vi "Find Workspace.vi"(6 "Pickup_Test_Number":dbl, 7 "Database Entry in":refnum<class "Database Entry.lvclass">, 8 "Error In":errorcluster, 9 "Assembly Type":string, 10 "Control In":T2={"I-O.lvclass"=refnum, "Gantry"=refnum, "Dispenser"="COM1"}, 11 "Carrier Tray in":refnum<class "Assembly Tray.lvclass">) -> (0 "Error Out":errorcluster, 1 "Workspace":T1, 2 "Control Out":T2={"I-O.lvclass"=refnum, "Gantry"=refnum, "Dispenser"="COM1"}, 3 "Carrier Tray Out":refnum<class "Assembly Tray.lvclass">, 5 "Database Entry out":refnum<class "Database Entry.lvclass">)   [LabVIEW 2021, in "Assembly Tray.lvclass"]
uses:
  Assembly Tray.lvclass
  C:/Users/HEP/Documents/GitHub/Gantry/UCSB-Gantry-HEP-main/Classes/Workspace/Fixture.lvclass
  Controller/Controllers.ctl
  Controller/I-O/I-O.lvclass
  C:/Program Files (x86)/Aerotech/A3200/LabVIEW/2010/Bin/Aerotech.A3200.dll
  Program Files (x86)/Aerotech/A3200/LabVIEW/2010/Bin/Aerotech.A3200.dll
  Workspace.ctl
  Assembly/Database Entry/Database Entry.lvclass
  Fixture.lvclass/Fixture.ctl
  Assembly Tray.lvclass/Assembly Tray.ctl
  Read Fixture ID.vi
  Read Position.vi
  Fixture.lvclass
  Controller/Controller.lvclass
panel:
  out "XYZTheta Centers":dbl[][](array[numeric])
  in  "output cluster 2":T1
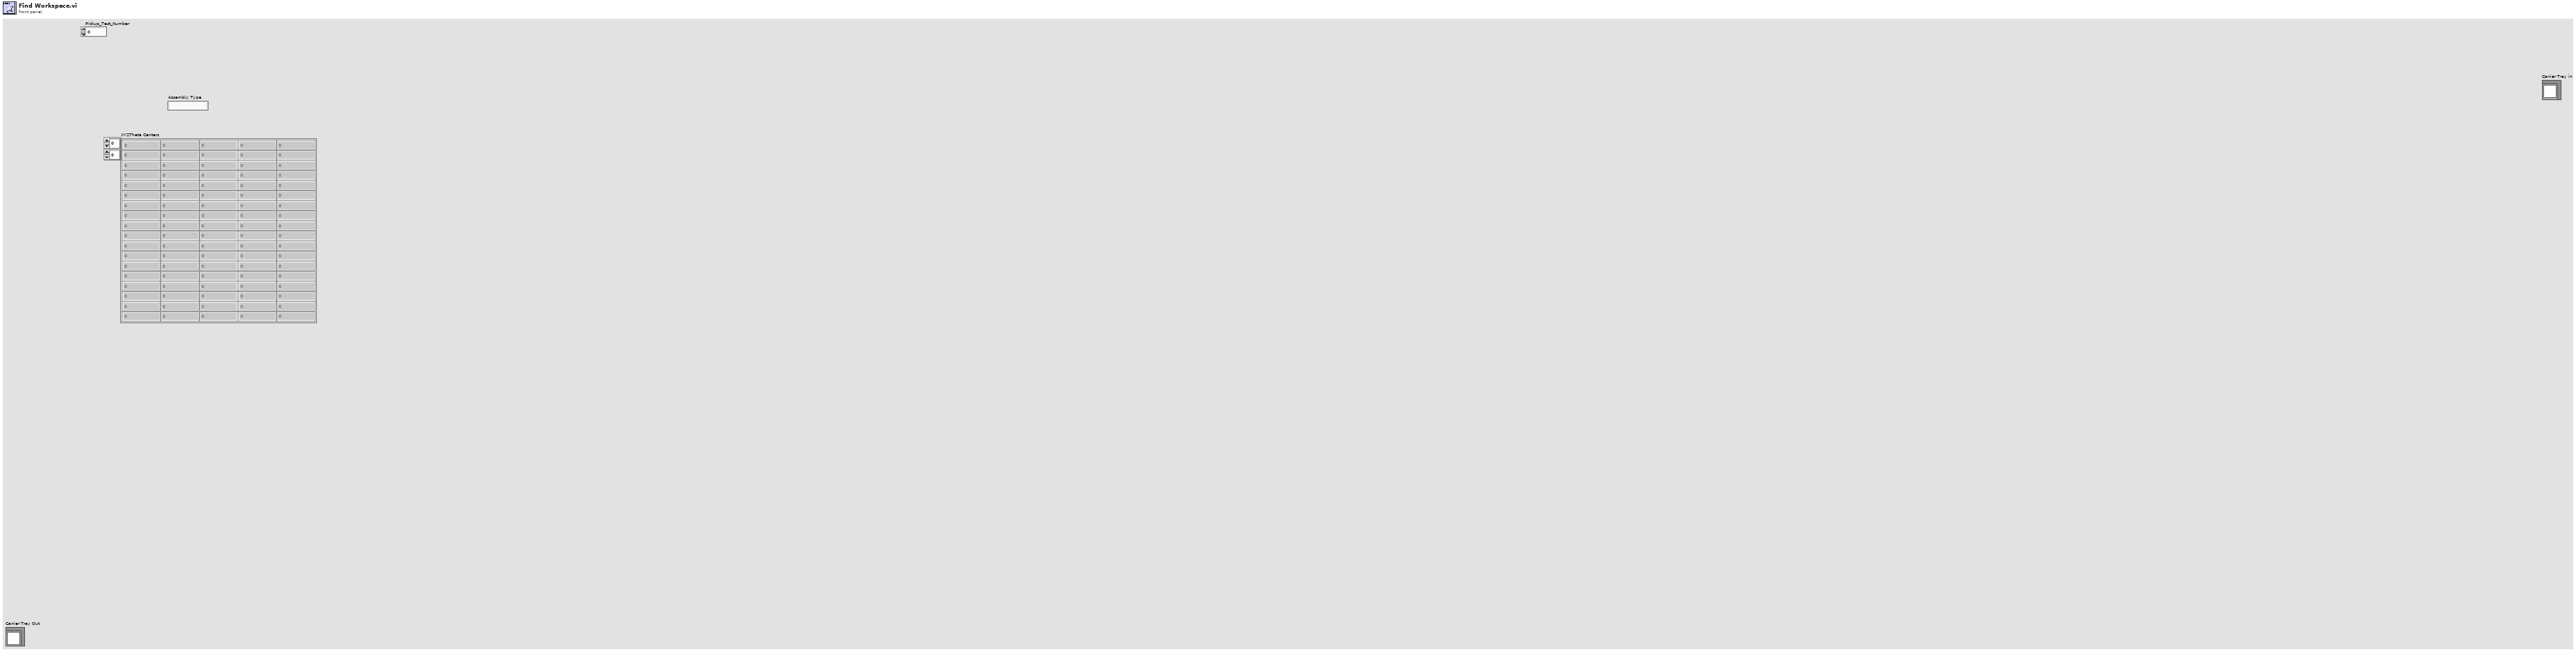
[diagram p1: front panel]
types:
  T1 = typedef "Fixture.lvclass/Workspace.ctl" = cluster{"XYZTheta":dbl[], "Workspace Valve":i32, "Workspace Sensor":i32, "Tray Number":i32, "Position":i32, "Assembly Type":string, "Numeric":dbl, "First Pos":i32}
  T2 = typedef "Controller.lvclass/Controllers.ctl" = cluster{"I-O.lvclass":refnum<class "I-O.lvclass">, "Gantry":refnum<k24>, "Dispenser":refnum<visa-resource-name>}
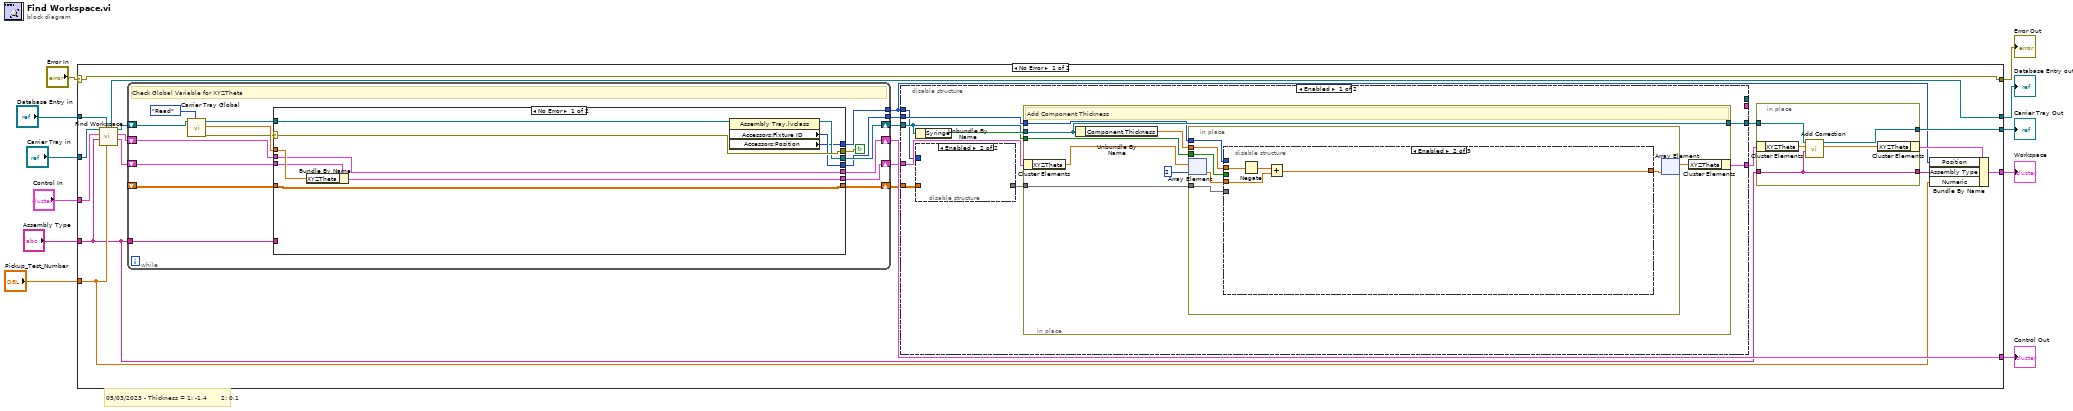
[diagram p0: block diagram]
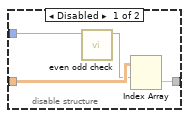
[diagram p2: hidden frame]
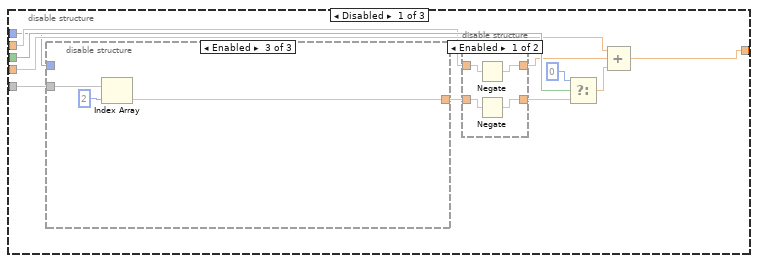
[diagram p3: hidden frame]
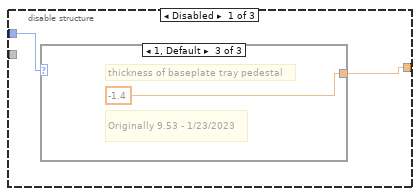
[diagram p4: hidden frame]
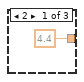
[diagram p5: hidden frame]
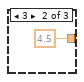
[diagram p6: hidden frame]
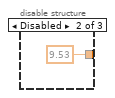
[diagram p7: hidden frame]
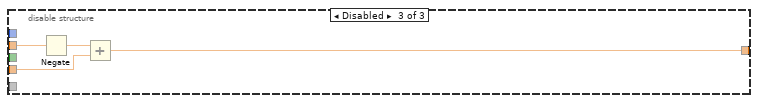
[diagram p9: hidden frame]
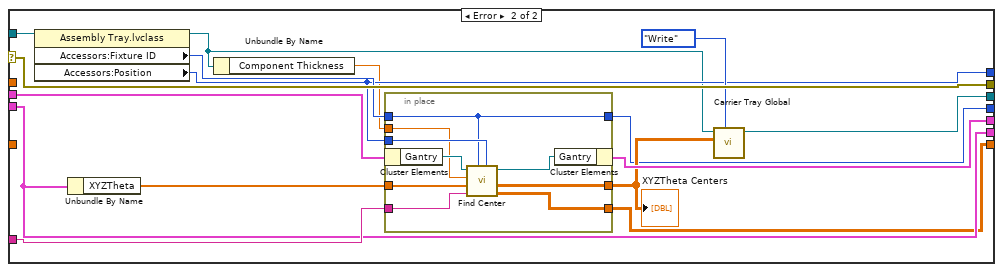
[diagram p11: hidden frame]
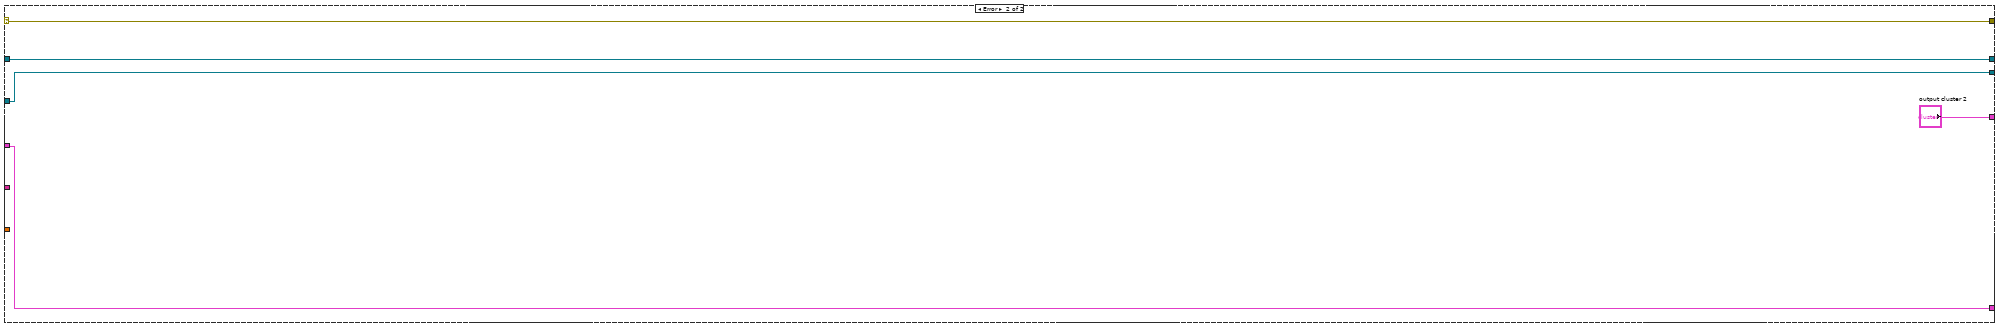
[diagram p12: hidden frame]
diagram:
  # "05/03/2023 - Thickness = 1: -1.4       2: 0.1"
  n1 = case shown="No Error" "Error In" {
    selector: "Error In" -> [w33 w156]
    tunnel: [w33 w156] -> w10
    tunnel: "Control In" -> [w32 w157]
    tunnel: [w30 w157] -> w8
    tunnel: "Carrier Tray in" -> [w31 w154]
    tunnel: [w18 "output cluster 2"] -> w6
    tunnel: [w20 w154] -> w5
    tunnel: "Assembly Type" -> [w12 _]
    tunnel: "Pickup_Test_Number" -> [w15 _]
    tunnel: "Database Entry in" -> [w14 w153]
    tunnel: [w13 w153] -> w1
    frame No Error {
      n2 = call-parent "Find Workspace.vi"("Pickup_Test_Number"=w15, "Database Entry in"=w14, "Assembly Type"=w12, "Control In"=w32, "Workspace In"=w31) -> (1:"Workspace Out"=w29:T1, "Control Out"=w28:T2, 3:"Workspace Out"=w25:refnum<class "Assembly Tray.lvclass">, "Database Entry out"=w13:refnum<class "Database Entry.lvclass">)  [unwired: 2 in, 1 out]
      n3 = while {
        shift-right: [w110] -> w27
        shift-left: w25 -> [w108]
        shift-right: [w112] -> w30
        shift-left: w28 -> [w113]
        shift-right: [w109] -> w26
        shift-left: w29 -> [w114]
        tunnel: w12 -> [w106]
        tunnel: [w105] -> w24
        shift-right: [w104] -> w23
        shift-left: _ -> [w103]
        tunnel: [w102] -> w16
        stop <- w116 continue-if-true
        # "Check Global Variable for XYZTheta"
        n4 = call "Carrier Tray Global.vi"("Action"=enum16{"Initialize", "Read", "Write"}."Read", "Carrier Tray.lvclass"=w108) -> ("error out"=w107:errorcluster, "XYZTheta out"=w115:dbl[], "Carrier Tray.lvclass 2"=w111:refnum<class "Assembly Tray.lvclass">)  [unwired: 7 in]
        n5 = case shown="No Error" w107 {
          selector: w107 -> [w127 w143]
          tunnel: [w127 w143] -> w116
          tunnel: w115 -> [w126 _]
          tunnel: [w125 w132] -> w109
          tunnel: w114 -> [w124 w132]
          tunnel: w113 -> [w123 w138]
          tunnel: [w123 w137] -> w112
          tunnel: w111 -> [w122 w140]
          tunnel: [w121 w142] -> w110
          tunnel: w106 -> [_ w134]
          tunnel: [w120 w133] -> w105
          tunnel: [w119 w131] -> w104
          tunnel: w103 -> [w119 _]
          tunnel: [w118 w130] -> w102
          frame No Error {
            n6 = Bundle By Name(cluster=w124, "XYZTheta"=w126) -> (w125:T1)
            n7 = property class="Assembly Tray.lvclass"(reference=w122) -> (reference out=w121:refnum<class "Assembly Tray.lvclass">, "Accessors:Fixture ID"=w120:i32, "Accessors:Position"=w118:i32)  [unwired: 1 in, 1 out]
          }
          frame Error {
            n8 = property class="Assembly Tray.lvclass"(reference=w140) -> (reference out=w129:refnum<class "Assembly Tray.lvclass">, "Accessors:Fixture ID"=w139:i32, "Accessors:Position"=w130:i32)  [unwired: 1 in, 1 out]
            n9 = Unbundle By Name(w132) -> ("XYZTheta"=w136:dbl[])
            n10 = Unbundle By Name(w129) -> ("Component Thickness"=w128:dbl)
            n11 = in-place {
              in-place-border: w139 -> [w146]
              in-place-border: w136 -> [w150]
              in-place-border: [w149] -> w135
              in-place-border: w134 -> [w148]
              in-place-border: w130 -> [w147]
              in-place-border: [w146] -> w133
              in-place-border: [w145] -> w131
              in-place-border: w128 -> [w144]
              n12 = in-place-cluster #1(w138) -> ("Gantry"=w152:refnum<k24>)
              n13 = call "Find Center.vi"("Position"=w147, "Tray Number"=w146, "Assembly Type"=w148, "XYZTheta"=w150, "component thickness"=w144, "Gantry In"=w152) -> ("Pedestal Heights"=w145:dbl[][], "XYZTheta Centers"=w149:dbl[][], "Gantry Out"=w151:refnum<k24>)  [unwired: 3 in]
              n14 = in-place-cluster #1("Gantry"=w151) -> (w137:T2)
            }
            "XYZTheta Centers" <- w135
            n15 = call "Carrier Tray Global.vi"("Action"=enum16{"Initialize", "Read", "Write"}."Write", "XYZTheta in"=w135, "Carrier Tray.lvclass"=w129) -> ("Carrier Tray.lvclass 2"=w142:refnum<class "Assembly Tray.lvclass">)  [unwired: 6 in, 2 out]
          }
        }
      }
      n16 = disable-structure shown="Enabled" {
        disable-tunnel: [_ w100] -> _
        disable-tunnel: [_ w101] -> _
        disable-tunnel: w27 -> [w47 w100]
        disable-tunnel: w26 -> [w46 w101]
        disable-tunnel: w24 -> [w44 _]
        disable-tunnel: w23 -> [w41 _]
        disable-tunnel: [w43 _] -> w22
        disable-tunnel: [w42 _] -> w21
        disable-tunnel: w16 -> [w39 _]
        frame Enabled {
          n17 = Unbundle By Name(w47) -> ("Syringe"=w45:bool)
          n18 = disable-structure shown="Enabled" {
            disable-tunnel: w41 -> [w51 _]
            disable-tunnel: [w50 _] -> w40
            disable-tunnel: w39 -> [w48 _]
            frame Disabled {
              n19 = call "even odd check.vi"("position"=w48) -> ("index"=w49:i32)  [unwired: 10 in]
              n20 = Index Array(array=w51, index (row)=w49) -> (element=w50:dbl[])  [unwired: 1 in]
            }
            frame Enabled {
            }
          }
          n21 = in-place {
            in-place-border: w47 -> [w57]
            in-place-border: [w57] -> w42
            in-place-border: w45 -> [w56]
            in-place-border: w44 -> [w54]
            in-place-border: w40 -> [w52]
            # "Add Component Thickness"
            n22 = in-place-cluster #2(w46) -> ("XYZTheta"=w55:dbl[])
            n23 = Unbundle By Name(w57) -> ("Component Thickness"=w58:dbl)
            n24 = in-place {
              in-place-border: w58 -> [w62]
              in-place-border: w56 -> [w64]
              in-place-border: w54 -> [w61]
              in-place-border: w52 -> [w60]
              n25 = in-place-array #3(w55, 2) -> (w63:dbl)
              n26 = disable-structure shown="Enabled" {
                disable-tunnel: [w76 w94 w98] -> w65
                disable-tunnel: w64 -> [w75 _ _]
                disable-tunnel: w63 -> [w72 w95 w99]
                disable-tunnel: w62 -> [w71 w93 w97]
                disable-tunnel: w61 -> [w67 _ _]
                disable-tunnel: w60 -> [w66 _ _]
                frame Disabled {
                  n27 = disable-structure shown="Enabled" {
                    disable-tunnel: [w78 9.53 w85] -> w69
                    disable-tunnel: w67 -> [w77 _ _]
                    disable-tunnel: w66 -> [_ _ w84]
                    frame Disabled {
                      n28 = case shown="1, Default" w77 {
                        tunnel: [4.4 4.5 -1.4] -> w78
                        frame 2 {
                        }
                        frame 3 {
                        }
                        frame 1, Default {
                          # "thickness of baseplate tray pedestal"
                          # "Originally 9.53 - 1/23/2023"
                        }
                      }
                    }
                    frame Disabled {
                    }
                    frame Enabled {
                      n29 = Index Array(array=w84, index=2) -> (element=w85:dbl)
                    }
                  }
                  n30 = disable-structure shown="Enabled" {
                    disable-tunnel: w71 -> [w89 w91]
                    disable-tunnel: [w88 w91] -> w70
                    disable-tunnel: w69 -> [w87 w90]
                    disable-tunnel: [w86 w90] -> w68
                    frame Enabled {
                      n31 = Negate(x=w89) -> (-x=w88:dbl)
                      n32 = Negate(x=w87) -> (-x=w86:dbl)
                    }
                    frame Disabled {
                    }
                  }
                  n33 = Select(t=0, s=w75, f=w68) -> (s? t:f=w73:dbl)
                  n34 = Compound Arithmetic op=ADD(w72, w70, w73) -> (w76:dbl)
                }
                frame Enabled {
                  n35 = Negate(x=w93) -> (-x=w92:dbl)
                  n36 = Add(x=w92, y=w95) -> (x+y=w94:dbl)
                }
                frame Disabled {
                  n37 = Negate(x=w97) -> (-x=w96:dbl)
                  n38 = Add(x=w96, y=w99) -> (x+y=w98:dbl)
                }
              }
              n39 = in-place-array #3(w65) -> (w59:dbl[])  [unwired: 1 out]
            }
            n40 = in-place-cluster #2("XYZTheta"=w59) -> (w43:T1)
          }
        }
        frame Disabled {
        }
      }
      n41 = in-place {
        in-place-border: [w38] -> w20
        in-place-border: w21 -> [w37]
        in-place-border: w12 -> [w34]
        in-place-border: [w34] -> w17
        n42 = in-place-cluster #4(w22) -> ("XYZTheta"=w36:dbl[])
        n43 = call "Add Correction.vi"("Assembly Type"=w34, "XYZTheta"=w36, "Carrier Tray in"=w37) -> ("XYZTheta Out"=w35:dbl[], "Carrier Tray out"=w38:refnum<class "Assembly Tray.lvclass">)  [unwired: 6 in, 1 out]
        n44 = in-place-cluster #4("XYZTheta"=w35) -> (w19:T1)
      }
      n45 = Bundle By Name(cluster=w19, "Position"=w16, "Assembly Type"=w17, "Numeric"=w15) -> (w18:T1)
    }
    frame Error {
    }
  }
  "Error Out" <- w10
  "Control Out" <- w8
  "Workspace" <- w6
  "Carrier Tray Out" <- w5
  "Database Entry out" <- w1
